vi "240126_Keyborad-Check.vi"(8 "error in (no error)":errorcluster, 10 "PlatMods":T1, 11 "VKey":T2) -> (0 "error out":errorcluster, 3 "String":string)   [LabVIEW 2014]
uses:
  <vilib>/event_ctls.llb/eventvkey.ctl
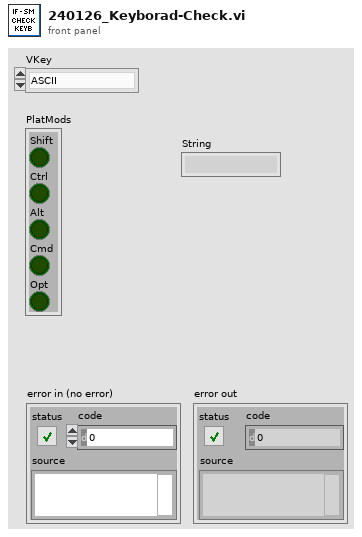
[diagram p1: front panel]
types:
  T1 = cluster{"Shift":bool, "Ctrl":bool, "Alt":bool, "Cmd":bool, "Opt":bool}
  T2 = typedef "eventvkey.ctl" = enum16{"ASCII", "Enter", "Return", "Shift", "Ctrl", "Alt", "Cmd", "Opt", "Caps", "NumLock", "Clear", "Break", "Up", "Down", "Left", "Right", "Insert", "Delete", "Home", "End", "PageUp", "PageDown", "Escape", "Help", "Pause", "ScrollLock", "F1", "F2", "F3", "F4", "F5", "F6", "F7", "F8", "F9", "F10", "F11", "F12", "F13", "F14", "F15", "F16", "F17", "F18", "F19", "F20", "F21", "F22", "F23", "F24", "Play", "VolumeUp", "VolumeDown", "Mute", "Two Byte Char"}
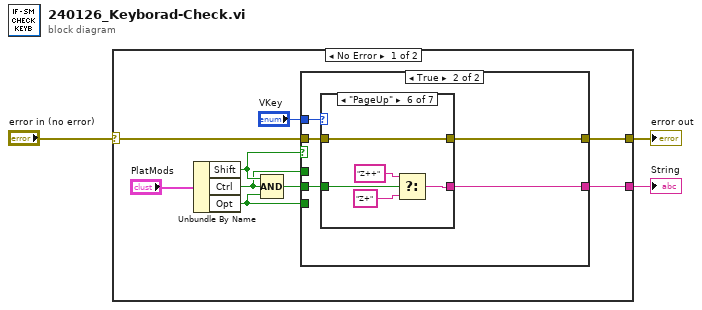
[diagram p0: block diagram]
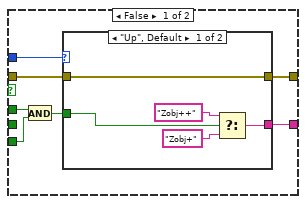
[diagram p2: hidden frame]
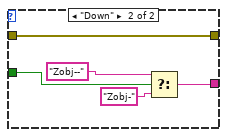
[diagram p3: hidden frame]
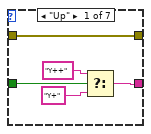
[diagram p4: hidden frame]
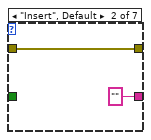
[diagram p5: hidden frame]
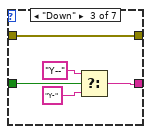
[diagram p6: hidden frame]
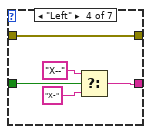
[diagram p7: hidden frame]
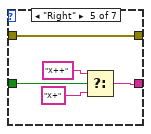
[diagram p8: hidden frame]
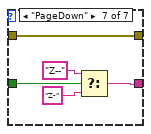
[diagram p9: hidden frame]
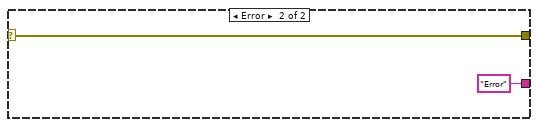
[diagram p10: hidden frame]
diagram:
  n1 = case shown="No Error" "error in (no error)" {
    selector: "error in (no error)" -> [w9 w68]
    tunnel: [w10 w68] -> w3
    tunnel: [w8 "Error"] -> w1
    frame No Error {
      n2 = Unbundle By Name("PlatMods") -> ("Shift"=w7:bool, "Ctrl"=w5:bool, "Opt"=w4:bool)
      n3 = Compound Arithmetic op=AND(w7, w5, w4) -> (w6:bool)
      n4 = case shown="True" w7 {
        tunnel: "VKey" -> [w19 w34]
        tunnel: [w17 w33] -> w10
        tunnel: w9 -> [w18 w32]
        tunnel: [w16 w31] -> w8
        tunnel: w6 -> [_ w30]
        tunnel: w5 -> [w15 _]
        tunnel: w4 -> [w14 _]
        frame False {
          n5 = And(x=w15, y=w14) -> (x .and. y?=w13:bool)
          n6 = case shown="\"Up\", Default" w19 {
            tunnel: [w24 w29] -> w17
            tunnel: [w22 w27] -> w16
            tunnel: w18 -> [w24 w29]
            tunnel: w13 -> [w20 w28]
            frame "Up", Default {
              n7 = Select(t="Zobj++", s=w20, f="Zobj+") -> (s? t:f=w22:string)
            }
            frame "Down" {
              n8 = Select(t="Zobj--", s=w28, f="Zobj-") -> (s? t:f=w27:string)
            }
          }
        }
        frame True {
          n9 = case shown="\"PageUp\"" w34 {
            tunnel: [w39 w41 w46 w51 w56 w61 w63] -> w33
            tunnel: w32 -> [w39 w41 w46 w51 w56 w61 w63]
            tunnel: [w35 "" w42 w49 w52 w58 w64] -> w31
            tunnel: w30 -> [w38 _ w43 w47 w55 w57 w62]
            frame "Up" {
              n10 = Select(t="Y++", s=w38, f="Y+") -> (s? t:f=w35:string)
            }
            frame "Insert", Default {
            }
            frame "Down" {
              n11 = Select(t="Y--", s=w43, f="Y-") -> (s? t:f=w42:string)
            }
            frame "Left" {
              n12 = Select(t="X--", s=w47, f="X-") -> (s? t:f=w49:string)
            }
            frame "Right" {
              n13 = Select(t="X++", s=w55, f="X+") -> (s? t:f=w52:string)
            }
            frame "PageUp" {
              n14 = Select(t="Z++", s=w57, f="Z+") -> (s? t:f=w58:string)
            }
            frame "PageDown" {
              n15 = Select(t="Z--", s=w62, f="Z-") -> (s? t:f=w64:string)
            }
          }
        }
      }
    }
    frame Error {
    }
  }
  "error out" <- w3
  "String" <- w1
